vi "Nodes Setting.vi"   [LabVIEW 2015]
uses:
  <vilib>/rvi/Emulation/niFpgaGetClockAttributes.vi
  <vilib>/rvi/Emulation/niFpgaSctlEmulationGetInTimedLoop.vi
  <vilib>/rvi/Emulation/niFpgaEmulationReportErrorSimple.vi
  <vilib>/rvi/eio/common/nirviEmuTemplateMethod_errors.vi
  <vilib>/rvi/Emulation/niFpgaCriticalErrorInLSC.vi
  <vilib>/eio/EIONode/EIONode.xnode
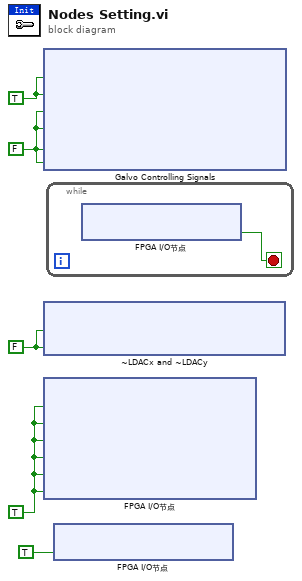
[diagram p0: block diagram]
diagram:
  w4 = TRUE ("IO Module\\DDCA_DIO8-15_WE")
  w3 = FALSE ("_LDACx")
  w2 = FALSE ("_CSx")
  w1 = TRUE ("_CLRx")
  n1 = xnode "Galvo Controlling Signals"("IO Module\\CLRx(DDCB_DIO0_WRITE)"=w1, "IO Module\\CLRy(DDCB_DIO1_WRITE)"=w1, "IO Module\\CSx(DDCB_DIO2_WRITE)"=w2, "IO Module\\CSy(DDCB_DIO3_WRITE)"=w2, "IO Module\\R_Wx(DDCB_DIO4_WRITE)"=w2, "IO Module\\R_Wy(DDCB_DIO5_WRITE)"=w2) -> ()  [unwired: 6 in, 6 out]
  n2 = xnode "~LDACx and ~LDACy"("IO Module\\LDAx(DDCB_DIO6_WRITE)"=w3, "IO Module\\LDAy(DDCB_DIO7_WRITE)"=w3) -> ()  [unwired: 2 in, 2 out]
  n3 = xnode "FPGA I/O节点"("IO Module\\DDCA_DIO8-15_WE"=w4, "IO Module\\DDCA_DIO16-23_WE"=w4, "IO Module\\DDCB_DIO8-15_WE"=w4, "IO Module\\DDCB_DIO16-23_WE"=w4, "IO Module\\DDCB_DIO0-7_WE"=w4, "IO Module\\DDCB_PFI_WE"=w4) -> ()  [unwired: 6 in, 6 out]
  n4 = while {
    stop <- w6 stop-if-true
    n5 = xnode "FPGA I/O节点"() -> ("IO Module IO Enabled"=w6:bool)  [unwired: 1 in, 1 out]
  }
  n6 = xnode "FPGA I/O节点"("IO Module\\DDCA_PFI_WE"=TRUE ("IO Module\\DDCA_DIO8-15_WE")) -> ()  [unwired: 1 in, 1 out]
